vi "General Linear Fit (LAR).vi"(0 "Y":dbl[](array[numeric]), 1 "covariance selector":T3(ring), 5 "H":dbl[][](array[numeric]), 7 "Weight":dbl[](array[numeric]), 9 "tolerance":dbl=0.0001, 13 "algorithm":T1 items=["SVD", "Givens", "Givens2", "Householder", "LU Decomposition", "Cholesky", "SVD for Rank Deficient H"]) -> (4 "Best Fit":dbl[](array[numeric]), 6 "Coefficients":dbl[](array[numeric]), 8 "Covariance":T2, 14 "residue":dbl, 15 "error":i32)   [LabVIEW 2010, in "NI_AALPro.lvlib"]
uses:
  NI_AALPro.lvlib
  RealMatrix.ctl
  General Linear Fit Algorithm.ctl
  Array To Matrix - RA2.vi
  NI_Matrix.lvlib
  lvanlys.dll
panel:
  # "LAR General Linear Fit"
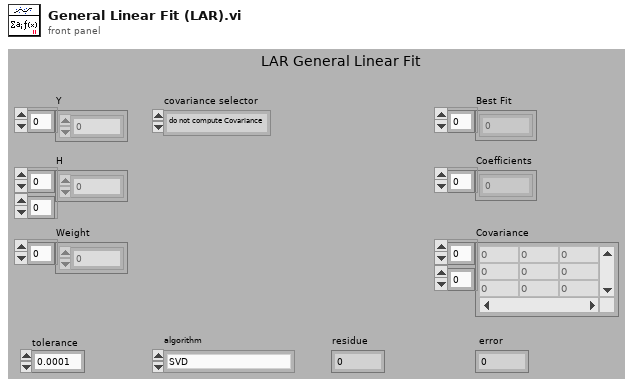
[diagram p1: front panel]
types:
  T1 = typedef "NI_AALPro.lvlib/General Linear Fit Algorithm.ctl" = u16
  T2 = typedef "NI_Matrix.lvlib/RealMatrix.ctl" = dbl[][]
  T3 = enum32{"do not compute Covariance", " compute Covariance"}
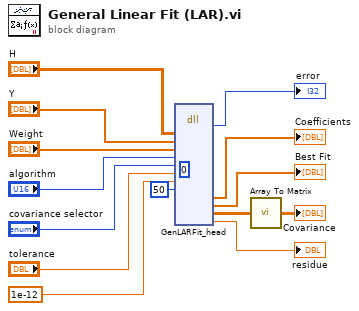
[diagram p0: block diagram]
diagram:
  (unwired) 0
  n1 = dll-call lib="C:/Program Files/National Instruments/LabVIEW 2010/resource/lvanlys.*" fn="GenLARFit_head"("H"="H", "Y Values"="Y", "Weight"="Weight", "algorithm"="algorithm", "covariance selector"="covariance selector", "tol"="tolerance", "absTol"=1e-12, "maxIter"=50) -> ("return type"=→"error":i32, "CoefH"=→"Coefficients":dbl[], "BestFitH"=→"Best Fit":dbl[], "CovarH"=w6:dbl[][], "mse"=→"residue":dbl)  [unwired: 9 in, 8 out]
  n2 = call-poly "Array To Matrix.vi"("Real 2D Array"=w6) -> ("Real Matrix"=→"Covariance":T2)
